vi "User Inputs Find Replace.vi"(11 "DesignRequest":T1) -> (3 "Find-Replace":cluster{"Find":string, "Replace":string}[](array[cluster]))   [LabVIEW 2012]
uses:
  Design Request.ctl
  Variable cluster.ctl
  Design Server.lvlib
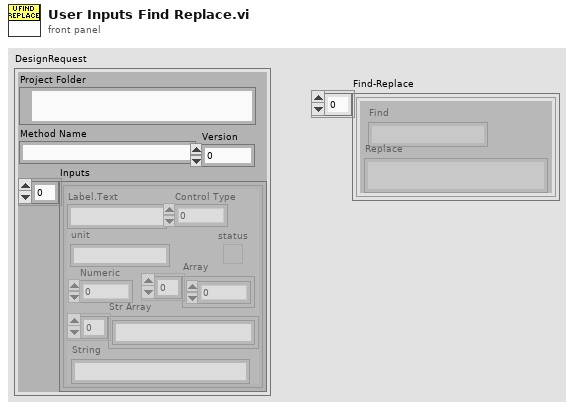
[diagram p1: front panel]
types:
  T1 = typedef "Design Server.lvlib/Design Request.ctl" = cluster{"Project Folder":path, "Method Name":string, "Inputs":T2, "Version":i32}
  T2 = typedef "Design Server.lvlib/Variable cluster.ctl" = cluster{"Label.Text":string, "Control Type":u32, "Numeric":dbl, "Array":dbl[], "status":bool, "Str Array":string[], "String":string, "unit":string}[]
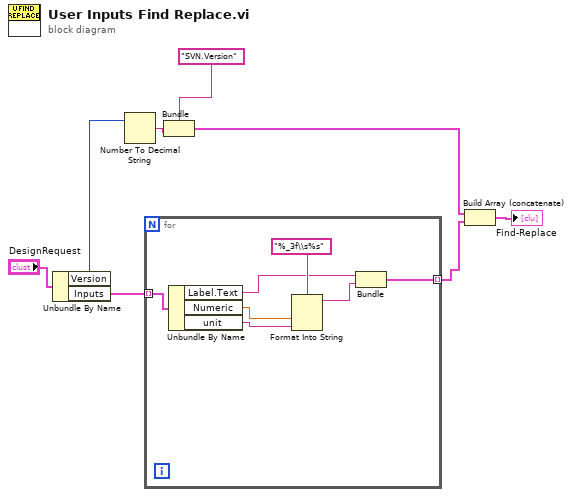
[diagram p0: block diagram]
diagram:
  n1 = Unbundle By Name("DesignRequest") -> ("Version"=w6:i32, "Inputs"=w4:T2)
  n2 = Number To Decimal String(number=w6) -> (decimal integer string=w7:string)  [unwired: 1 in]
  n3 = for {
    tunnel: w4 -> [w15] mode=indexing
    tunnel: [w9] -> w3 mode=indexing
    n4 = Unbundle By Name(w15) -> ("Label.Text"=w10:string, "Numeric"=w13:dbl, "unit"=w12:string)
    n5 = Format Into String(format string="%_3f\\s%s", w13, w12) -> (resulting string=w11:string)  [unwired: 2 in, 1 out]
    n6 = Bundle("Label.Text"=w10, w11) -> (w9:cluster{"Label.Text":string, string})  [unwired: 1 in]
  }
  n7 = Bundle("Version string"="SVN.Version", w7) -> (w2:cluster{"Version string":string, string})  [unwired: 1 in]
  n8 = Build Array (concatenate)(w2, w3) -> (→"Find-Replace":cluster{"Label.Text":string, string}[])
